vi "Query DUT SIM Slot Catalog.vi"(8 "error in (no error)":errorcluster, 10 "DUT (\"DUT1\")":string="DUT1", 11 "VISA resource name":refnum<visa-resource-name>) -> (0 "error out":errorcluster, 2 "DUT SIM Slots":string, 3 "VISA resource name out":refnum<visa-resource-name>)   [LabVIEW 2015, in "Rohde&Schwarz CMXP Base.lvlib"]
doc: "Queries all SIM slots of the inactive DUT. For each SIM slot, the number and the slot name are returned:\n\n{<SimSlotNo>, <SimProfileName>}1, {...}2, ...\n\nAttribute:\n-\n\nRemote-control command:\nCATalog:DUT:PROFile:SIMSlot?"
uses:
  <instrlib>/Rohde&Schwarz CMXP Base/Rohde&Schwarz CMXP Base.lvlib
  <instrlib>/Rohde&Schwarz CMXP Base/Private/rsidr_core.llb/rsidr_core.lvlib
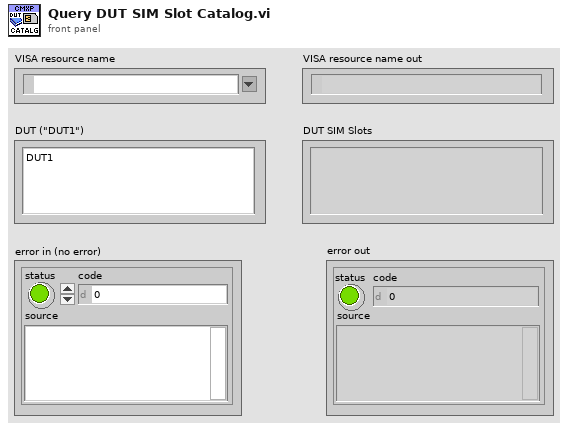
[diagram p1: front panel]
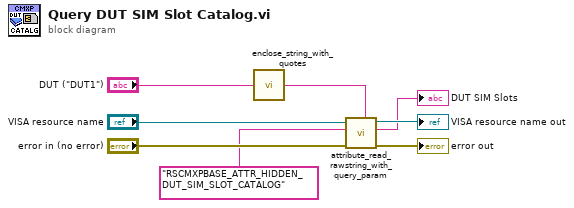
[diagram p0: block diagram]
diagram:
  n1 = call <instrlib>:"enclose_string_with_quotes.vi"("String to enclose"="DUT (\"DUT1\")") -> ("String out"=w2:string)  [unwired: 4 in]
  n2 = call <instrlib>:"attribute_read_rawstring_with_query_param.vi"("Query Parameter (None)"=w2, "error in"="error in (no error)", "Attribute ID"="RSCMXPBASE_ATTR_HIDDEN_DUT_SIM_SLOT_CATALOG", "VISA resource name"="VISA resource name") -> ("error out"=→"error out":errorcluster, "RawString out"=→"DUT SIM Slots":string, "VISA resource name out"=→"VISA resource name out":refnum<visa-resource-name>)  [unwired: 5 in]
